vi "加密解密字符串（XOR 数组）.vi"(8 "error in (no error)":errorcluster caption="错误输入（无错误）", 9 "密钥":string, 10 "模式":enum16{"加密", "解密"}(ring), 11 "输入字符串":string) -> (0 "error out":errorcluster caption="错误输出", 3 "输出字符串":string)   [LabVIEW 2012]
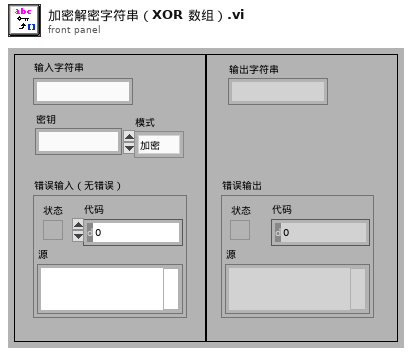
[diagram p1: front panel]
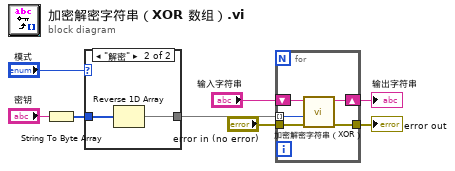
[diagram p0: block diagram]
diagram:
  n1 = String To Byte Array(string="密钥") -> (unsigned byte array=w1:u8[])
  n2 = case shown="\"解密\"" "模式" {
    tunnel: [w9 w11] -> w3
    tunnel: w1 -> [w9 w10]
    frame "加密", Default {
    }
    frame "解密" {
      n3 = Reverse 1D Array(array=w10) -> (reversed array=w11:u8[])
    }
  }
  n4 = for {
    tunnel: w3 -> [w16] mode=indexing
    shift-right: [w14] -> w7
    shift-left: "输入字符串" -> [w15]
    tunnel: "error in (no error)" -> [w13]
    tunnel: [w12] -> w5
    n5 = call "加密解密字符串（XOR）.vi"("error in (no error)"=w13, "密钥"=w16, "输入字符串"=w15) -> ("error out"=w12:errorcluster, "输出字符串"=w14:string)  [unwired: 7 in]
  }
  "输出字符串" <- w7
  "error out" <- w5
